vi "reward_behavior_michelle_visjitter_conswinAdapt_enticefx_TSLog_VF.vi"() -> ()   [LabVIEW 2019]
doc: "The myRIO Project template acquires acceleration data from the onboard accelerometer and displays the changes of acceleration values in a waveform chart."
uses:
  <vilib>/myRIO/Common/Instrument Driver Framework/Utilities/typedefs/Generic FPGA Reference.ctl
  <vilib>/myRIO/Common/Instrument Driver Framework/Utilities/typedefs/myRIO v1.0 Reference.ctl
  <vilib>/myRIO/Common/Instrument Driver Framework/Utilities/typedefs/Hardware Version Enum.ctl
  <vilib>/myRIO/Common/Instrument Driver Framework/Utilities/typedefs/myRIO Generic Hardware Reference.ctl
  <vilib>/userdefined/High Color/nirio_resource_hc.ctl
  <vilib>/myRIO/Common/Instrument Driver Framework/Utilities/vis/Is FPGA Ref Available.vi
  <vilib>/myRIO/Common/Instrument Driver Framework/myRIO v1.0/Encoder/typedefs/Encoder Signal Mode.ctl
  <vilib>/myRIO/Common/Instrument Driver Framework/myRIO v1.0/Encoder/typedefs/Encoder Channels Enum.ctl
  <vilib>/myRIO/Instrument Drivers/Onboard IO/Encoder/typedefs/Encoder Reference.ctl
  <vilib>/myRIO/Instrument Drivers/Onboard IO/Encoder/Encoder.lvlib
  <vilib>/myRIO/Instrument Drivers/Onboard IO/Encoder/vis/Read.vi
  <vilib>/myRIO/Common/Instrument Driver Framework/myRIO v1.0/Encoder/typedefs/Encoder Configuration v1.0.ctl
  <vilib>/myRIO/Common/Instrument Driver Framework/myRIO v1.0/Encoder/vis/myRIO v1.1 Open Encoder.vi
  <vilib>/myRIO/Common/Instrument Driver Framework/myRIO v1.0/Encoder/vis/myRIO v1.0 Configure Encoder.vi
  <vilib>/myRIO/Instrument Drivers/Onboard IO/Encoder/vis/myRIO Encoder Open.xnode
  <vilib>/myRIO/Express VI/Onboard IO/Encoder/Encoder Express VI.xnode
  <vilib>/myRIO/Express VI/Onboard IO/DI/DI Express VI.xnode
  <vilib>/myRIO/Instrument Drivers/Onboard IO/DIO/vis/Read.vi
  <vilib>/myRIO/Instrument Drivers/Onboard IO/DIO/DIO.lvlib
  <vilib>/myRIO/Common/Instrument Driver Framework/myRIO v1.0/DIO/typedefs/DIO Channels Enum.ctl
  <vilib>/myRIO/Common/Instrument Driver Framework/myRIO v1.0/DIO/typedefs/DIO Channels List.ctl
  <vilib>/myRIO/Instrument Drivers/Onboard IO/DIO/typedefs/DIO Reference.ctl
  <vilib>/myRIO/Instrument Drivers/Onboard IO/DIO/vis/myRIO DIO Open.xnode
  <vilib>/myRIO/Common/Instrument Driver Framework/myRIO v1.0/DIO/vis/myRIO v1.1 Open DIO.vi
  <vilib>/myRIO/Instrument Drivers/Onboard IO/DIO/vis/Write.vi
  <vilib>/myRIO/Express VI/Onboard IO/DO/DO Express VI.xnode
  <vilib>/myRIO/Common/Instrument Driver Framework/myRIO v1.0/Encoder/typedefs/Encoder Count Direction Enum.ctl
  <vilib>/Analysis/Matrix/Datatypes/RealMatrix.ctl
  <vilib>/Analysis/Matrix/NI_Matrix.lvlib
panel:
  out "GetVidFrame":i32
  out "VidTS":dbl[][](array[numeric])
  out "VidFrameClock":i32
  out "EntTS":dbl[][](array[numeric])
  out "TimeLag":dbl
  out "Lag2":dbl
  out "TestTime":dbl
  out "RewTS":dbl[][](array[numeric])
  out "ConsTS":dbl[][](array[numeric])
  out "LickTS":dbl[][](array[numeric])
  out "ContrastChoice":dbl
  out "Its":i32
  out "BurstCriteria":dbl
  out "LickBurst 2":bool
  out "LickBurst":bool
  out "Enticements":i32
  in  "Entice":bool
  out "Misses":i32
  out "GoAhead":bool
  out "TimeOutDuration":i32
  out "ActiveTime":dbl
  out "ConsumptionGo":bool=TRUE
  out "Consumption_Period":i32
  out "Watch_Display":bool=TRUE
  in  "Give reward":bool
  out "Timings":dbl[](array[numeric])
  out "ISI":dbl
  out "ISI start time":dbl
  out "Time_out":bool=TRUE
  out "Time since lick":dbl
  out "Time of last lick":dbl
  out "Rewarded trials":dbl[](array[numeric])
  out "Rewards":u16
  out "Active Trial":bool
  out "Array temp2":T1
  out "Stimuli Loaded":bool
  out "Stim_ID":dbl[](array[numeric])
  out "Reward_mat":dbl[](array[numeric])
  out "Reward":bool=TRUE
  out "Frame clock":i32
  out "Licks":u32
  out "Lick":bool
  out "Time":dbl
  out "Stop":bool
  in  "Frames to collect":u32
  out "Overflow?":bool
  out "Counter Value":i32
  out "Velocity":dbl
  out "Velocity Plot":dbl[](graph)
  out "Velocity array":dbl[](array[numeric])
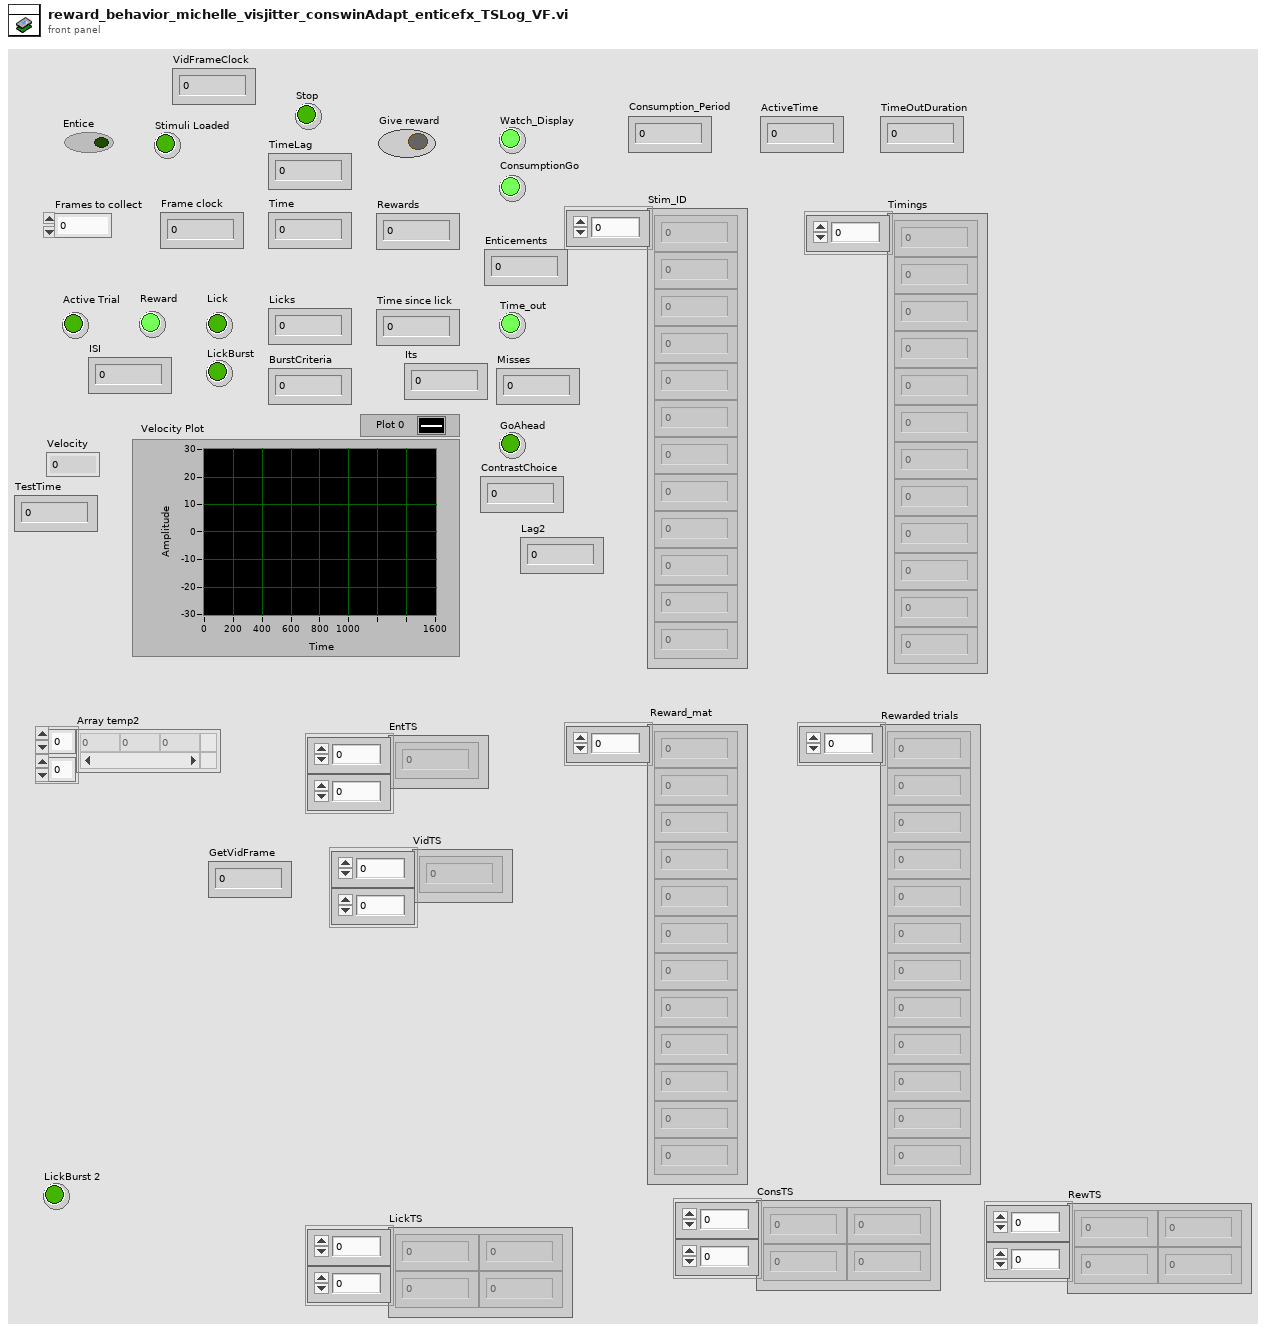
[diagram p1: front panel]
types:
  T1 = typedef "NI_Matrix.lvlib/RealMatrix.ctl" = dbl[][]
  T2 = typedef "Encoder.lvlib/Encoder Reference.ctl" = cluster{"myRIO Reference":T3, "Encoder Channels Enum":T7}
  T3 = typedef "myRIO Generic Hardware Reference.ctl" = cluster{"myRIO Model":T4, "myRIO Hardware Reference":T5}
  T4 = typedef "Hardware Version Enum.ctl" = enum16{"Unknown", "myRIO-1900", "myRIO-1950", "roboRIO", "NI ELVIS RIO CM", "ELVIS III"}
  T5 = typedef "myRIO v1.0 Reference.ctl" = cluster{"Generic FPGA Reference":T6, "Allow multiple opens":bool}
  T6 = typedef "Generic FPGA Reference.ctl" = refnum<k20>
  T7 = typedef "Encoder Channels Enum.ctl" = enum16{"Not Connected", "C/ENC0", "C/ENC1", "A/ENC", "A/ENC0", "A/ENC1", "A/ENC2", "A/ENC3", "A/ENC4", "A/ENC5", "A/ENC6", "A/ENC7", "A/ENC8", "A/ENC9", "B/ENC", "B/ENC0", "B/ENC1", "B/ENC2", "B/ENC3", "B/ENC4", "B/ENC5", "B/ENC6", "B/ENC7", "B/ENC8", "B/ENC9", "DIO/ENC0", "DIO/ENC1", "DIO/ENC2", "DIO/ENC3", "DIO/ENC4"}
  T8 = typedef "Encoder Signal Mode.ctl" = enum16{"Quadrature phase signal", "Step and direction signal"}
  T9 = typedef "nirio_resource_hc.ctl" = tag
  T10 = typedef "DIO.lvlib/DIO Reference.ctl" = cluster{"myRIO Reference":T3, "DIO Channels List":T11}
  T11 = typedef "DIO Channels List.ctl" = T12[]
  T12 = typedef "DIO Channels Enum.ctl" = enum16{"Not Connected", "C/DIO0", "C/DIO1", "C/DIO2", "C/DIO3", "C/DIO4", "C/DIO5", "C/DIO6", "C/DIO7", "A/DIO0", "A/DIO1", "A/DIO2", "A/DIO3", "A/DIO4", "A/DIO5", "A/DIO6", "A/DIO7", "A/DIO8", "A/DIO9", "A/DIO10", "A/DIO11", "A/DIO12", "A/DIO13", "A/DIO14", "A/DIO15", "A/DIO16", "A/DIO17", "A/DIO18", "A/DIO19", "B/DIO0", "B/DIO1", "B/DIO2", "B/DIO3", "B/DIO4", "B/DIO5", "B/DIO6", "B/DIO7", "B/DIO8", "B/DIO9", "B/DIO10", "B/DIO11", "B/DIO12", "B/DIO13", "B/DIO14", "B/DIO15", "B/DIO16", "B/DIO17", "B/DIO18", "B/DIO19", "LED0", "LED1", "LED2", "LED3", "Button0", "DIO/DIO0", "DIO/DIO1", "DIO/DIO2", "DIO/DIO3", "DIO/DIO4", "DIO/DIO5", "DIO/DIO6", "DIO/DIO7", "DIO/DIO8", "DIO/DIO9", "SPI/CS0", "SPI/CS1", "SPI/CS2", "SPI/CS3", "LED RADIO (Green)", "LED RADIO (Red)", "LED COMM (Green)", "LED COMM (Red)", "LED MODE (Green)", "LED MODE (Red)"}
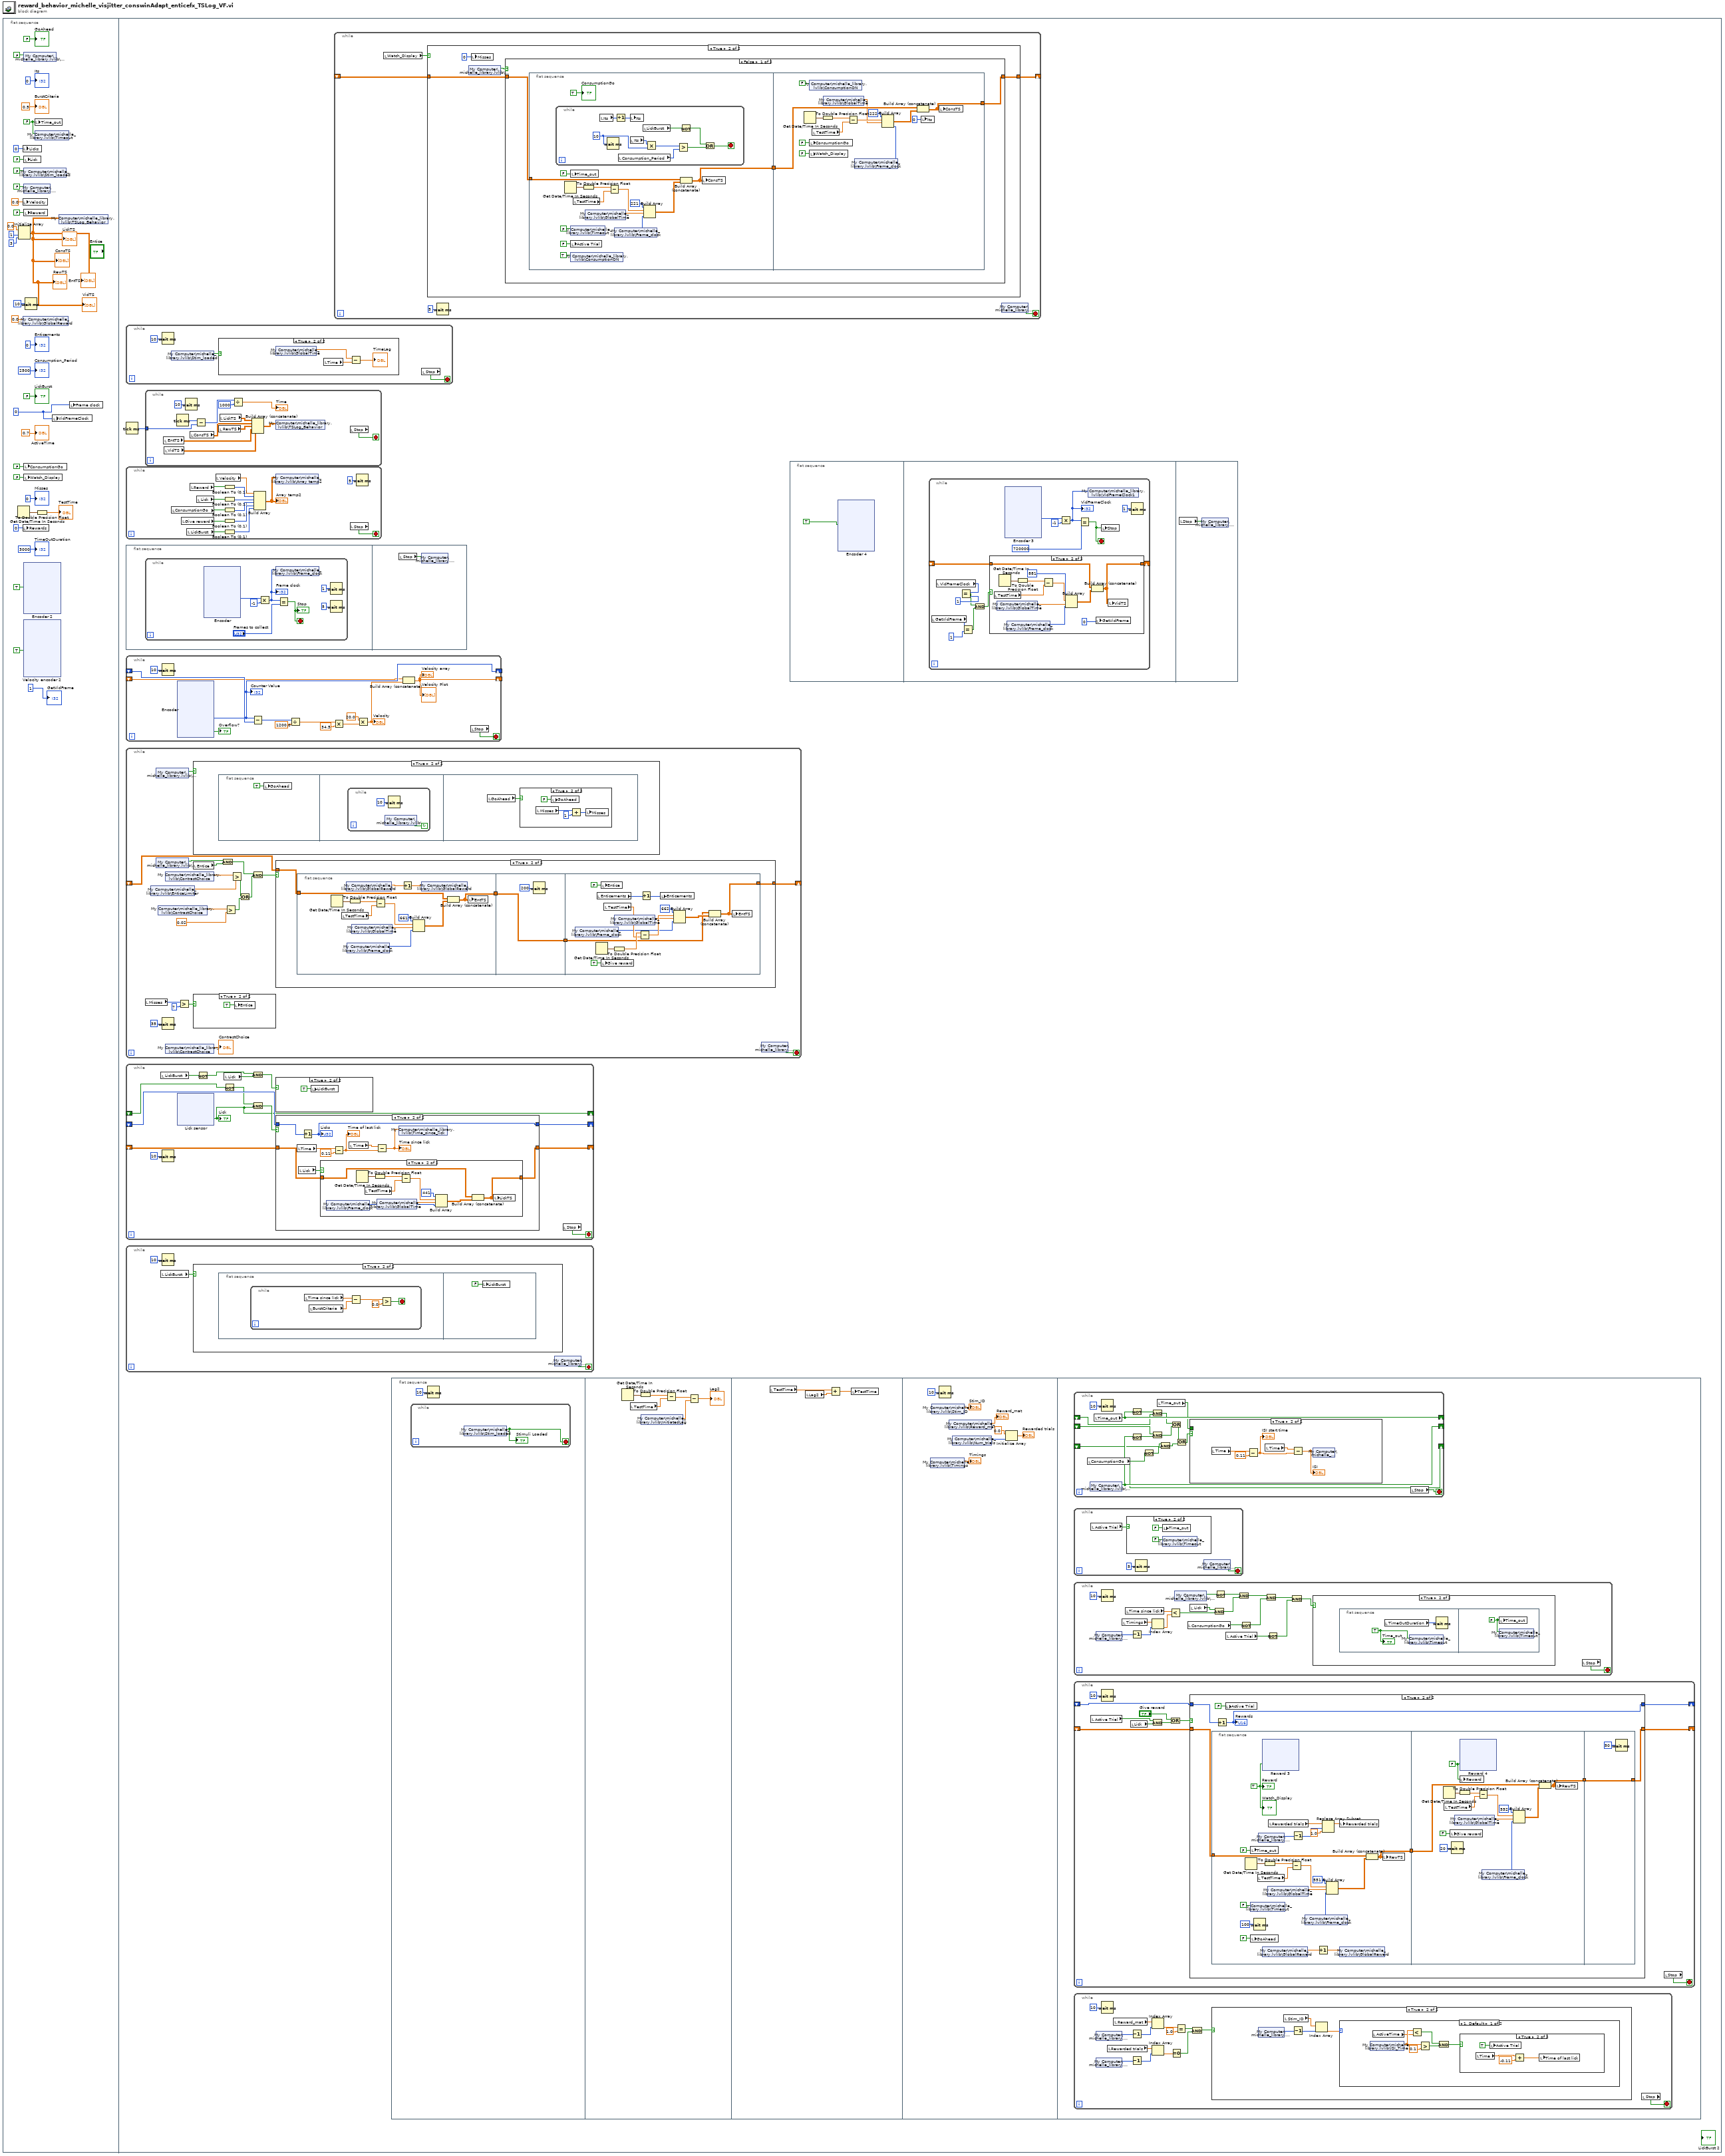
[diagram p0: block diagram]
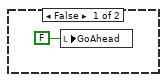
[diagram p7: hidden frame]
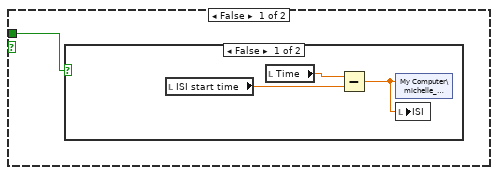
[diagram p13: hidden frame]
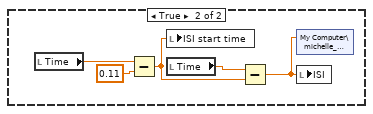
[diagram p14: hidden frame]
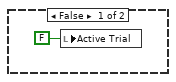
[diagram p15: hidden frame]
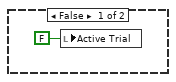
[diagram p16: hidden frame]
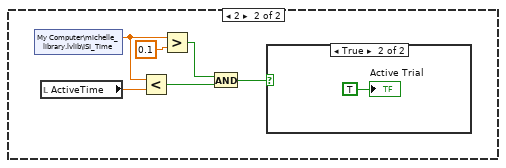
[diagram p17: hidden frame]
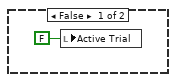
[diagram p18: hidden frame]
diagram:
  n1 = flat-sequence {
    frame #0 {
      w21 = FALSE ("Time_out")
      w3 = u32 0 ("Frames")
      n2 = Get Date/Time In Seconds() -> (seconds since 1Jan1904=w5:timestamp)
      n3 = Initialize Array(0.0, 1, 3) -> (w2:dbl[][])
      "LickTS" <- w2
      "ConsTS" <- w2
      "RewTS" <- w2
      "EntTS" <- w2
      "VidTS" <- w2
      n4 = local write "Licks"(u32 0 ("Licks")) -> ()
      n5 = local write "Velocity"(0.0 ("Velocity")) -> ()
      n6 = shared-variable "My Computer\\michelle_library.lvlib\\GlobalReward"(0.0) -> ()  [unwired: 1 in, 1 out]
      n7 = local write "Rewards"(u16 0 ("Rewards")) -> ()
      n8 = shared-variable "My Computer\\michelle_library.lvlib\\Display"(FALSE ("Display")) -> ()  [unwired: 1 in, 1 out]
      n9 = local write "Lick"(FALSE ("Lick")) -> ()
      n10 = shared-variable "My Computer\\michelle_library.lvlib\\Stim_loaded"(FALSE ("Stim_loaded")) -> ()  [unwired: 1 in, 1 out]
      n11 = shared-variable "My Computer\\michelle_library.lvlib\\Stop"(FALSE ("Stop")) -> ()  [unwired: 1 in, 1 out]
      n12 = local write "Reward"(FALSE ("Give reward")) -> ()
      n13 = local write "ConsumptionGo"(FALSE ("ConsumptionGo")) -> ()
      n14 = local write "Watch_Display"(FALSE ("Watch_Display")) -> ()
      n15 = xnode "Encoder 2"("Reset Counter"=TRUE) -> ()  [unwired: 1 in, 4 out]
      n16 = xnode "Velocity encoder 2"("Reset Counter"=TRUE) -> ()  [unwired: 1 in, 4 out]
      n17 = Wait (ms)(milliseconds to wait=u32 10) -> ()  [unwired: 1 out]
      n18 = local write "Time_out"(w21) -> ()
      n19 = shared-variable "My Computer\\michelle_library.lvlib\\Timeout"(w21) -> ()  [unwired: 1 in, 1 out]
      n20 = To Double Precision Float(number=w5) -> (double precision float=→"TestTime":dbl)
      n21 = local write "VidFrameClock"(w3) -> ()
      n22 = shared-variable "My Computer\\michelle_library.lvlib\\TSLog_Behavior"(w2) -> ()  [unwired: 1 in, 1 out]
      n23 = local write "Frame clock"(w3) -> ()
      "Consumption_Period" <- 2500
      "ActiveTime" <- 0.7
      "TimeOutDuration" <- 3000
      "GoAhead" <- FALSE
      "Misses" <- 0
      "Enticements" <- 0
      "LickBurst" <- FALSE
      "BurstCriteria" <- 0.5
      "Its" <- 0
      "GetVidFrame" <- 1
    }
    frame #1 {
      n24 = while {
        stop <- w248 stop-if-true
        n25 = Wait (ms)(milliseconds to wait=u32 10) -> ()  [unwired: 1 out]
        n26 = shared-variable "My Computer\\michelle_library.lvlib\\Stim_loaded"() -> (w249:bool)  [unwired: 1 in, 1 out]
        n27 = case shown="True" w249 {
          frame False {
          }
          frame True {
            n28 = shared-variable "My Computer\\michelle_library.lvlib\\GlobalTime"() -> (w250:dbl)  [unwired: 1 in, 1 out]
            n29 = local read "Time"() -> (w251:dbl)
            n30 = Subtract(x=w250, y=w251) -> (x-y=→"TimeLag":dbl)
          }
        }
        n31 = local read "Stop"() -> (w248:bool)
      }
      n32 = Tick Count (ms)() -> (millisecond timer value=w125:u32)
      n33 = while {
        stop <- w385 stop-if-true
        n34 = local read "ConsumptionGo"() -> (w383:bool)
        n35 = local read "Give reward"() -> (w382:bool)
        n36 = local read "LickBurst"() -> (w379:bool)
        n37 = local read "Reward"() -> (w390:bool)
        n38 = local read "Lick"() -> (w391:bool)
        n39 = local read "Velocity"() -> (w389:dbl)
        n40 = Boolean To (0,1)(Boolean=w390) -> (0, 1=w388:i16)
        n41 = Boolean To (0,1)(Boolean=w391) -> (0, 1=w387:i16)
        n42 = Boolean To (0,1)(Boolean=w383) -> (0, 1=w381:i16)
        n43 = Boolean To (0,1)(Boolean=w382) -> (0, 1=w380:i16)
        n44 = Boolean To (0,1)(Boolean=w379) -> (0, 1=w378:i16)
        n45 = Build Array(w389, w388, w387, w381, w380, w378) -> (w384:T1)
        "Array temp2" <- w384
        n46 = shared-variable "My Computer\\michelle_library.lvlib\\Array temp2"(w384) -> ()  [unwired: 1 in, 1 out]
        n47 = local read "Stop"() -> (w385:bool)
        n48 = Wait (ms)(milliseconds to wait=u32 5) -> ()  [unwired: 1 out]
      }
      n49 = flat-sequence {
        frame #0 {
          n50 = while {
            stop <- w634 stop-if-true
            n51 = xnode "Encoder"() -> ("Counter Value"=w638:i32)  [unwired: 2 in, 3 out]
            n52 = Multiply(x=w638, y=-1) -> (x*y=w633:i32)
            "Frame clock" <- w633
            n53 = shared-variable "My Computer\\michelle_library.lvlib\\Frame_clock"(w633) -> ()  [unwired: 1 in, 1 out]
            n54 = Equal?(x=w633, y="Frames to collect") -> (x = y?=w634:bool)
            "Stop" <- w634
            n55 = Wait (ms)(milliseconds to wait=u32 1) -> ()  [unwired: 1 out]
            n56 = Wait (ms)(milliseconds to wait=u32 5) -> ()  [unwired: 1 out]
          }
        }
        frame #1 {
          n57 = local read "Stop"() -> (w686:bool)
          n58 = shared-variable "My Computer\\michelle_library.lvlib\\Stop"(w686) -> ()  [unwired: 1 in, 1 out]
        }
      }
      n59 = while {
        shift-right: [w773] -> _
        shift-left: _ -> [w774]
        shift-right: [w765] -> _
        shift-left: _ -> [w764]
        stop <- w763 stop-if-true
        n60 = Wait (ms)(milliseconds to wait=u32 10) -> ()  [unwired: 1 out]
        n61 = xnode "Encoder"() -> ("Counter Value"=w773:i32, "Overflow?"=→"Overflow?":bool)  [unwired: 2 in, 2 out]
        "Counter Value" <- w773
        n62 = Subtract(x=w773, y=w774) -> (x-y=w766:i32)
        n63 = Divide(x=w766, y=1200.0 ("600")) -> (x/y=w771:dbl)
        n64 = Multiply(x=w771, y=34.5) -> (x*y=w769:dbl)
        n65 = Multiply(x=20.0, y=w769) -> (x*y=w767:dbl)
        "Velocity" <- w767
        n66 = Build Array (concatenate)(w764, w767) -> (w765:dbl[])
        "Velocity Plot" <- w765
        "Velocity array" <- w765
        n67 = local read "Stop"() -> (w763:bool)
      }
      n68 = while {
        shift-right: [w268] -> _
        shift-left: _ -> [w269]
        stop <- w281 stop-if-true
        n69 = local read "Misses"() -> (w279:i32)
        n70 = shared-variable "My Computer\\michelle_library.lvlib\\EnticeLimiter"() -> (w267:dbl)  [unwired: 1 in, 1 out]
        n71 = shared-variable "My Computer\\michelle_library.lvlib\\Display"() -> (w280:bool)  [unwired: 1 in, 1 out]
        n72 = shared-variable "My Computer\\michelle_library.lvlib\\Display"() -> (w276:bool)  [unwired: 1 in, 1 out]
        n73 = shared-variable "My Computer\\michelle_library.lvlib\\ContrastChoice"() -> (w263:dbl)  [unwired: 1 in, 1 out]
        n74 = Wait (ms)(milliseconds to wait=35) -> ()  [unwired: 1 out]
        n75 = shared-variable "My Computer\\michelle_library.lvlib\\ContrastChoice"() -> (w272:dbl)  [unwired: 1 in, 1 out]
        n76 = shared-variable "My Computer\\michelle_library.lvlib\\ContrastChoice"() -> (→"ContrastChoice":dbl)  [unwired: 1 in, 1 out]
        n77 = Greater?(x=w279, y=7) -> (0:w277:bool)
        n78 = case shown="True" w280 {
          frame False {
            n79 = local write "GoAhead"(FALSE) -> ()
          }
          frame True {
            n80 = flat-sequence {
              frame #0 {
                n81 = local write "GoAhead"(TRUE) -> ()
              }
              frame #1 {
                n82 = while {
                  stop <- w319 continue-if-true
                  n83 = shared-variable "My Computer\\michelle_library.lvlib\\Display"() -> (w319:bool)  [unwired: 1 in, 1 out]
                  n84 = Wait (ms)(milliseconds to wait=10) -> ()  [unwired: 1 out]
                }
              }
              frame #2 {
                n85 = local read "GoAhead"() -> (w320:bool)
                n86 = case shown="True" w320 {
                  frame False {
                  }
                  frame True {
                    n87 = local read "Misses"() -> (w324:i32)
                    n88 = local write "GoAhead"(FALSE) -> ()
                    n89 = Add(x=w324, y=1) -> (x+y=w322:i32)
                    n90 = local write "Misses"(w322) -> ()
                  }
                }
              }
            }
          }
        }
        n91 = local read "Entice"() -> (w275:bool)
        n92 = case shown="True" w277 {
          frame False {
          }
          frame True {
            n93 = local write "Entice"(TRUE) -> ()
          }
        }
        n94 = And(x=w276, y=w275) -> (x .and. y?=w273:bool)
        n95 = Greater?(x=w263, y=0.02) -> (0:w264:bool)
        n96 = Greater?(x=w272, y=w267) -> (0:w265:bool)
        n97 = Or(x=w265, y=w264) -> (x .or. y?=w266:bool)
        n98 = And(x=w273, y=w266) -> (x .and. y?=w271:bool)
        n99 = case shown="True" w271 {
          tunnel: w269 -> [w282 w286]
          tunnel: [w282 w283] -> w268
          frame False {
          }
          frame True {
            n100 = flat-sequence {
              tunnel: w286 -> [w289]
              tunnel: [w288] -> w285
              tunnel: w285 -> [w299]
              tunnel: [w299] -> w284
              tunnel: w284 -> [w303]
              tunnel: [w302] -> w283
              frame #0 {
                n101 = Get Date/Time In Seconds() -> (seconds since 1Jan1904=w296:timestamp)
                n102 = local read "TestTime"() -> (w291:dbl)
                n103 = shared-variable "My Computer\\michelle_library.lvlib\\GlobalReward"() -> (w298:dbl)  [unwired: 1 in, 1 out]
                n104 = shared-variable "My Computer\\michelle_library.lvlib\\Frame_clock"() -> (w287:u32)  [unwired: 1 in, 1 out]
                n105 = To Double Precision Float(number=w296) -> (double precision float=w295:dbl)
                n106 = shared-variable "My Computer\\michelle_library.lvlib\\GlobalTime"() -> (w290:dbl)  [unwired: 1 in, 1 out]
                n107 = Subtract(x=w295, y=w291) -> (x-y=w294:dbl)
                n108 = Increment(x=w298) -> (x+1=w297:dbl)
                n109 = Build Array(661, w294, w290, w287) -> (w293:T1)
                n110 = shared-variable "My Computer\\michelle_library.lvlib\\GlobalReward"(w297) -> ()  [unwired: 1 in, 1 out]
                n111 = Build Array (concatenate) ("Build Matrix")(w289, w293) -> (w288:T1)
                n112 = local write "EntTS"(w288) -> ()
              }
              frame #1 {
                n113 = Wait (ms)(milliseconds to wait=200) -> ()  [unwired: 1 out]
              }
              frame #2 {
                n114 = shared-variable "My Computer\\michelle_library.lvlib\\Frame_clock"() -> (w301:u32)  [unwired: 1 in, 1 out]
                n115 = Get Date/Time In Seconds() -> (seconds since 1Jan1904=w310:timestamp)
                n116 = local read "Enticements"() -> (w312:i32)
                n117 = local write "Entice"(FALSE) -> ()
                n118 = local write "Give reward"(TRUE) -> ()
                n119 = local read "TestTime"() -> (w304:dbl)
                n120 = To Double Precision Float(number=w310) -> (double precision float=w309:dbl)
                n121 = shared-variable "My Computer\\michelle_library.lvlib\\GlobalTime"() -> (w305:dbl)  [unwired: 1 in, 1 out]
                n122 = Subtract(x=w309, y=w304) -> (x-y=w308:dbl)
                n123 = Increment(x=w312) -> (x+1=w311:i32)
                n124 = local write "Enticements"(w311) -> ()
                n125 = Build Array(662, w308, w305, w301) -> (w307:T1)
                n126 = Build Array (concatenate) ("Build Matrix")(w303, w307) -> (w302:T1)
                n127 = local write "EntTS"(w302) -> ()
              }
            }
          }
        }
        n128 = shared-variable "My Computer\\michelle_library.lvlib\\Stop"() -> (w281:bool)  [unwired: 1 in, 1 out]
      }
      n129 = while {
        shift-right: [w699] -> _
        shift-left: _ -> [w698]
        shift-right: [w693] -> _
        shift-left: _ -> [w696]
        shift-right: [w687] -> _
        shift-left: _ -> [w688]
        stop <- w697 stop-if-true
        n130 = local read "LickBurst"() -> (w690:bool)
        n131 = Wait (ms)(milliseconds to wait=u32 10) -> ()  [unwired: 1 out]
        n132 = xnode "Lick sensor"() -> ("C/DIO1 (DIO1)"=w693:bool)  [unwired: 1 in, 1 out]
        "Lick" <- w693
        n133 = Not(x=w690) -> (.not. x?=w689:bool)
        n134 = Not(x=w696) -> (.not. x?=w695:bool)
        n135 = local read "Lick"() -> (w691:bool)
        n136 = And(x=w689, y=w691) -> (x .and. y?=w692:bool)
        n137 = And(x=w695, y=w693) -> (x .and. y?=w694:bool)
        n138 = case shown="True" w692 {
          frame False {
          }
          frame True {
            n139 = local write "LickBurst"(TRUE) -> ()
          }
        }
        n140 = case shown="True" w694 {
          tunnel: [w706 w716] -> w699
          tunnel: w698 -> [w706 w715]
          tunnel: w688 -> [w702 w707]
          tunnel: [w702 w709] -> w687
          frame False {
            n141 = local read "Time of last lick"() -> (w704:dbl)
            n142 = local read "Time"() -> (w705:dbl)
            n143 = Subtract(x=w705, y=w704) -> (x-y=w703:dbl)
            n144 = shared-variable "My Computer\\michelle_library.lvlib\\Time_since_lick"(w703) -> ()  [unwired: 1 in, 1 out]
            n145 = local write "Time since lick"(w703) -> ()
          }
          frame True {
            n146 = local read "Time"() -> (w712:dbl)
            n147 = local read "Lick"() -> (w708:bool)
            n148 = Increment(x=w715) -> (x+1=w716:u32)
            "Licks" <- w716
            n149 = case shown="True" w708 {
              tunnel: w707 -> [w717 w723]
              tunnel: [w717 w722] -> w709
              frame False {
              }
              frame True {
                n150 = shared-variable "My Computer\\michelle_library.lvlib\\Frame_clock"() -> (w718:u32)  [unwired: 1 in, 1 out]
                n151 = Get Date/Time In Seconds() -> (seconds since 1Jan1904=w725:timestamp)
                n152 = local read "TestTime"() -> (w720:dbl)
                n153 = To Double Precision Float(number=w725) -> (double precision float=w721:dbl)
                n154 = shared-variable "My Computer\\michelle_library.lvlib\\GlobalTime"() -> (w719:dbl)  [unwired: 1 in, 1 out]
                n155 = Subtract(x=w721, y=w720) -> (x-y=w726:dbl)
                n156 = Build Array(441, w726, w719, w718) -> (w727:T1)
                n157 = Build Array (concatenate) ("Build Matrix")(w723, w727) -> (w722:T1)
                n158 = local write "LickTS"(w722) -> ()
              }
            }
            n159 = Subtract(x=w712, y=0.11) -> (x-y=w710:dbl)
            "Time of last lick" <- w710
            n160 = local read "Time"() -> (w714:dbl)
            n161 = Subtract(x=w714, y=w710) -> (x-y=w713:dbl)
            "Time since lick" <- w713
            n162 = shared-variable "My Computer\\michelle_library.lvlib\\Time_since_lick"(w713) -> ()  [unwired: 1 in, 1 out]
          }
        }
        n163 = local read "Stop"() -> (w697:bool)
      }
      n164 = while {
        stop <- w255 stop-if-true
        n165 = local read "LickBurst"() -> (w253:bool)
        n166 = Wait (ms)(milliseconds to wait=u32 10) -> ()  [unwired: 1 out]
        n167 = case shown="True" w253 {
          frame False {
          }
          frame True {
            n168 = flat-sequence {
              frame #0 {
                n169 = while {
                  stop <- w258 stop-if-true
                  n170 = local read "Time since lick"() -> (w259:dbl)
                  n171 = local read "BurstCriteria"() -> (w260:dbl)
                  n172 = Subtract(x=w259, y=w260) -> (x-y=w256:dbl)
                  n173 = Greater?(x=w256, y=0.0) -> (0:w258:bool)
                }
              }
              frame #1 {
                n174 = local write "LickBurst"(FALSE) -> ()
              }
            }
          }
        }
        n175 = shared-variable "My Computer\\michelle_library.lvlib\\Stop"() -> (w255:bool)  [unwired: 1 in, 1 out]
      }
      n176 = while {
        tunnel: w125 -> [w834]
        stop <- w832 stop-if-true
        n177 = local read "EntTS"() -> (w824:dbl[][])
        n178 = local read "VidTS"() -> (w823:dbl[][])
        n179 = Tick Count (ms)() -> (millisecond timer value=w835:u32)
        n180 = Wait (ms)(milliseconds to wait=u32 10) -> ()  [unwired: 1 out]
        n181 = local read "ConsTS"() -> (w827:dbl[][])
        n182 = Subtract(x=w835, y=w834) -> (x-y=w831:u32)
        n183 = local read "RewTS"() -> (w826:dbl[][])
        n184 = local read "LickTS"() -> (w828:dbl[][])
        n185 = Divide(x=w831, y=u32 1000) -> (x/y=→"Time":dbl)
        n186 = Build Array (concatenate) ("Build Matrix")(w828, w827, w826, w824, w823) -> (w825:T1)
        n187 = shared-variable "My Computer\\michelle_library.lvlib\\TSLog_Behavior"(w825) -> ()  [unwired: 1 in, 1 out]
        n188 = local read "Stop"() -> (w832:bool)
      }
      n189 = while {
        shift-right: [w325] -> _
        shift-left: _ -> [w326]
        stop <- w329 stop-if-true
        n190 = local read "Watch_Display"() -> (w328:bool)
        n191 = case shown="True" w328 {
          tunnel: w326 -> [w330 w332]
          tunnel: [w330 w331] -> w325
          frame False {
          }
          frame True {
            n192 = shared-variable "My Computer\\michelle_library.lvlib\\Display"() -> (w334:bool)  [unwired: 1 in, 1 out]
            n193 = local write "Misses"(0) -> ()
            n194 = case shown="False" w334 {
              tunnel: w332 -> [w337 w377]
              tunnel: [w335 w377] -> w331
              frame False {
                n195 = flat-sequence {
                  tunnel: w337 -> [w341]
                  tunnel: [w340] -> w336
                  tunnel: w336 -> [w367]
                  tunnel: [w366] -> w335
                  frame #0 {
                    n196 = while {
                      stop <- w356 stop-if-true
                      w357 = 10
                      n197 = local read "Its"() -> (w361:i32)
                      n198 = Wait (ms)(milliseconds to wait=w357) -> ()  [unwired: 1 out]
                      n199 = Increment(x=w361) -> (x+1=w360:i32)
                      n200 = local read "Consumption_Period"() -> (w354:i32)
                      n201 = local write "Its"(w360) -> ()
                      n202 = local read "Its"() -> (w358:i32)
                      n203 = local read "LickBurst"() -> (w362:bool)
                      n204 = Multiply(x=w358, y=w357) -> (x*y=w355:i32)
                      n205 = Greater?(x=w355, y=w354) -> (0:w353:bool)
                      n206 = Not(x=w362) -> (.not. x?=w359:bool)
                      n207 = Or(x=w359, y=w353) -> (x .or. y?=w356:bool)
                    }
                    n208 = Get Date/Time In Seconds() -> (seconds since 1Jan1904=w346:timestamp)
                    n209 = local write "Time_out"(FALSE) -> ()
                    n210 = shared-variable "My Computer\\michelle_library.lvlib\\Timeout"(FALSE) -> ()  [unwired: 1 in, 1 out]
                    n211 = local write "Active Trial"(FALSE) -> ()
                    n212 = shared-variable "My Computer\\michelle_library.lvlib\\ConsumptionON"(TRUE) -> ()  [unwired: 1 in, 1 out]
                    n213 = local read "TestTime"() -> (w343:dbl)
                    n214 = To Double Precision Float(number=w346) -> (double precision float=w344:dbl)
                    n215 = shared-variable "My Computer\\michelle_library.lvlib\\GlobalTime"() -> (w339:dbl)  [unwired: 1 in, 1 out]
                    n216 = Subtract(x=w344, y=w343) -> (x-y=w347:dbl)
                    n217 = shared-variable "My Computer\\michelle_library.lvlib\\Frame_clock"() -> (w338:u32)  [unwired: 1 in, 1 out]
                    n218 = Build Array(221, w347, w339, w338) -> (w342:T1)
                    n219 = Build Array (concatenate) ("Build Matrix")(w341, w342) -> (w340:T1)
                    n220 = local write "ConsTS"(w340) -> ()
                    "ConsumptionGo" <- TRUE
                  }
                  frame #1 {
                    n221 = Get Date/Time In Seconds() -> (seconds since 1Jan1904=w371:timestamp)
                    n222 = shared-variable "My Computer\\michelle_library.lvlib\\ConsumptionON"(FALSE) -> ()  [unwired: 1 in, 1 out]
                    n223 = local write "ConsumptionGo"(FALSE ("ConsumptionGo")) -> ()
                    n224 = local write "Watch_Display"(FALSE ("Watch_Display")) -> ()
                    n225 = local read "TestTime"() -> (w368:dbl)
                    n226 = To Double Precision Float(number=w371) -> (double precision float=w369:dbl)
                    n227 = shared-variable "My Computer\\michelle_library.lvlib\\GlobalTime"() -> (w364:dbl)  [unwired: 1 in, 1 out]
                    n228 = Subtract(x=w369, y=w368) -> (x-y=w372:dbl)
                    n229 = shared-variable "My Computer\\michelle_library.lvlib\\Frame_clock"() -> (w363:u32)  [unwired: 1 in, 1 out]
                    n230 = Build Array(222, w372, w364, w363) -> (w365:T1)
                    n231 = Build Array (concatenate) ("Build Matrix")(w367, w365) -> (w366:T1)
                    n232 = local write "Its"(0) -> ()
                    n233 = local write "ConsTS"(w366) -> ()
                  }
                }
              }
              frame True {
              }
            }
          }
        }
        n234 = Wait (ms)(milliseconds to wait=u32 5) -> ()  [unwired: 1 out]
        n235 = shared-variable "My Computer\\michelle_library.lvlib\\Stop"() -> (w329:bool)  [unwired: 1 in, 1 out]
      }
      n236 = flat-sequence {
        frame #0 {
          n237 = while {
            stop <- w393 stop-if-true
            n238 = shared-variable "My Computer\\michelle_library.lvlib\\Stim_loaded"() -> (w393:bool)  [unwired: 1 in, 1 out]
            "Stimuli Loaded" <- w393
          }
          n239 = Wait (ms)(milliseconds to wait=u32 10) -> ()  [unwired: 1 out]
        }
        frame #1 {
          n240 = Get Date/Time In Seconds() -> (seconds since 1Jan1904=w399:timestamp)
          n241 = local read "TestTime"() -> (w398:dbl)
          n242 = To Double Precision Float(number=w399) -> (double precision float=w397:dbl)
          n243 = shared-variable "My Computer\\michelle_library.lvlib\\InitiatedLag"() -> (w396:dbl)  [unwired: 1 in, 1 out]
          n244 = Subtract(x=w397, y=w398) -> (x-y=w394:dbl)
          n245 = Subtract(x=w394, y=w396) -> (x-y=→"Lag2":dbl)
        }
        frame #2 {
          n246 = local read "TestTime"() -> (w400:dbl)
          n247 = local read "Lag2"() -> (w401:dbl)
          n248 = Add(x=w400, y=w401) -> (x+y=w402:dbl)
          n249 = local write "TestTime"(w402) -> ()
        }
        frame #3 {
          n250 = shared-variable "My Computer\\michelle_library.lvlib\\Timings"() -> (→"Timings":dbl[])  [unwired: 1 in, 1 out]
          n251 = shared-variable "My Computer\\michelle_library.lvlib\\Stim_ID"() -> (→"Stim_ID":dbl[])  [unwired: 1 in, 1 out]
          n252 = Wait (ms)(milliseconds to wait=u32 10) -> ()  [unwired: 1 out]
          n253 = shared-variable "My Computer\\michelle_library.lvlib\\Reward_mat"() -> (→"Reward_mat":dbl[])  [unwired: 1 in, 1 out]
          n254 = shared-variable "My Computer\\michelle_library.lvlib\\Num_trials"() -> (w406:u32)  [unwired: 1 in, 1 out]
          n255 = Initialize Array(0.0 ("element"), w406) -> (→"Rewarded trials":dbl[])
        }
        frame #4 {
          n256 = while {
            shift-right: [w452] -> _
            shift-left: _ -> [w450]
            shift-right: [w448] -> _
            shift-left: _ -> [w447]
            shift-right: [w442] -> _
            shift-left: _ -> [w440]
            stop <- w453 stop-if-true
            n257 = local read "ConsumptionGo"() -> (w442:bool)
            n258 = shared-variable "My Computer\\michelle_library.lvlib\\Display"() -> (w448:bool)  [unwired: 1 in, 1 out]
            n259 = local read "Time_out"() -> (w452:bool)
            n260 = Wait (ms)(milliseconds to wait=u32 10) -> ()  [unwired: 1 out]
            n261 = Not(x=w452) -> (.not. x?=w451:bool)
            n262 = Not(x=w448) -> (.not. x?=w446:bool)
            n263 = Not(x=w442) -> (.not. x?=w443:bool)
            n264 = And(x=w451, y=w450) -> (x .and. y?=w445:bool)
            n265 = And(x=w447, y=w446) -> (x .and. y?=w441:bool)
            n266 = local read "Time_out"() -> (w449:bool)
            n267 = And(x=w440, y=w443) -> (x .and. y?=w439:bool)
            n268 = Or(x=w445, y=w441) -> (x .or. y?=w438:bool)
            n269 = Or(x=w438, y=w439) -> (x .or. y?=w437:bool)
            n270 = case shown="True" w437 {
              tunnel: w449 -> [w454 _]
              frame False {
                n271 = case shown="False" w454 {
                  frame False {
                    n272 = local read "ISI start time"() -> (w457:dbl)
                    n273 = local read "Time"() -> (w456:dbl)
                    n274 = Subtract(x=w456, y=w457) -> (x-y=w455:dbl)
                    n275 = shared-variable "My Computer\\michelle_library.lvlib\\ISI"(w455) -> ()  [unwired: 1 in, 1 out]
                    n276 = local write "ISI"(w455) -> ()
                  }
                  frame True {
                    n277 = local read "Time"() -> (w462:dbl)
                    n278 = Subtract(x=w462, y=0.11) -> (x-y=w459:dbl)
                    n279 = local write "ISI start time"(w459) -> ()
                    n280 = local read "Time"() -> (w460:dbl)
                    n281 = Subtract(x=w460, y=w459) -> (x-y=w458:dbl)
                    n282 = shared-variable "My Computer\\michelle_library.lvlib\\ISI"(w458) -> ()  [unwired: 1 in, 1 out]
                    n283 = local write "ISI"(w458) -> ()
                  }
                }
              }
              frame True {
                n284 = local read "Time"() -> (w467:dbl)
                n285 = Subtract(x=w467, y=0.11) -> (x-y=w464:dbl)
                "ISI start time" <- w464
                n286 = local read "Time"() -> (w465:dbl)
                n287 = Subtract(x=w465, y=w464) -> (x-y=w463:dbl)
                "ISI" <- w463
                n288 = shared-variable "My Computer\\michelle_library.lvlib\\ISI"(w463) -> ()  [unwired: 1 in, 1 out]
              }
            }
            n289 = local read "Stop"() -> (w453:bool)
          }
          n290 = while {
            stop <- w412 stop-if-true
            n291 = local read "Active Trial"() -> (w411:bool)
            n292 = case shown="True" w411 {
              frame False {
              }
              frame True {
                n293 = local write "Time_out"(FALSE) -> ()
                n294 = shared-variable "My Computer\\michelle_library.lvlib\\Timeout"(FALSE) -> ()  [unwired: 1 in, 1 out]
              }
            }
            n295 = Wait (ms)(milliseconds to wait=5) -> ()  [unwired: 1 out]
            n296 = shared-variable "My Computer\\michelle_library.lvlib\\Stop"() -> (w412:bool)  [unwired: 1 in, 1 out]
          }
          n297 = while {
            stop <- w433 stop-if-true
            n298 = shared-variable "My Computer\\michelle_library.lvlib\\Trial"() -> (w423:u32)  [unwired: 1 in, 1 out]
            n299 = Wait (ms)(milliseconds to wait=u32 10) -> ()  [unwired: 1 out]
            n300 = local read "Timings"() -> (w425:dbl[])
            n301 = local read "Time since lick"() -> (w432:dbl)
            n302 = Decrement(x=w423) -> (x-1=w422:u32)
            n303 = Index Array(array=w425, index=w422) -> (element=w424:dbl)
            n304 = Less?(x=w432, y=w424) -> (x < y?=w431:bool)
            n305 = shared-variable "My Computer\\michelle_library.lvlib\\Display"() -> (w428:bool)  [unwired: 1 in, 1 out]
            n306 = local read "ConsumptionGo"() -> (w420:bool)
            n307 = local read "Lick"() -> (w430:bool)
            n308 = And(x=w430, y=w431) -> (x .and. y?=w426:bool)
            n309 = Not(x=w428) -> (.not. x?=w427:bool)
            n310 = local read "Active Trial"() -> (w415:bool)
            n311 = And(x=w427, y=w426) -> (x .and. y?=w419:bool)
            n312 = Not(x=w420) -> (.not. x?=w421:bool)
            n313 = And(x=w419, y=w421) -> (x .and. y?=w417:bool)
            n314 = Not(x=w415) -> (.not. x?=w418:bool)
            n315 = And(x=w417, y=w418) -> (x .and. y?=w416:bool)
            n316 = case shown="True" w416 {
              frame False {
              }
              frame True {
                n317 = flat-sequence {
                  frame #0 {
                    w435 = TRUE
                    n318 = local read "TimeOutDuration"() -> (w434:i32)
                    n319 = shared-variable "My Computer\\michelle_library.lvlib\\Timeout"(w435) -> ()  [unwired: 1 in, 1 out]
                    n320 = Wait (ms)(milliseconds to wait=w434) -> ()  [unwired: 1 out]
                    "Time_out" <- w435
                  }
                  frame #1 {
                    w436 = FALSE ("Timeout")
                    n321 = local write "Time_out"(w436) -> ()
                    n322 = shared-variable "My Computer\\michelle_library.lvlib\\Timeout"(w436) -> ()  [unwired: 1 in, 1 out]
                  }
                }
              }
            }
            n323 = local read "Stop"() -> (w433:bool)
          }
          n324 = while {
            shift-right: [w514] -> _
            shift-left: _ -> [w513]
            shift-right: [w506] -> _
            shift-left: _ -> [w507]
            stop <- w516 stop-if-true
            n325 = local read "Active Trial"() -> (w511:bool)
            n326 = Wait (ms)(milliseconds to wait=u32 10) -> ()  [unwired: 1 out]
            n327 = local read "Lick"() -> (w512:bool)
            n328 = And(x=w511, y=w512) -> (x .and. y?=w510:bool)
            n329 = Or(x="Give reward", y=w510) -> (x .or. y?=w509:bool)
            n330 = case shown="True" w509 {
              tunnel: [w518 w525] -> w514
              tunnel: w513 -> [w518 w524]
              tunnel: w507 -> [w517 w522]
              tunnel: [w517 w521] -> w506
              frame False {
              }
              frame True {
                n331 = flat-sequence {
                  tunnel: w522 -> [w531]
                  tunnel: [w528] -> w519
                  tunnel: [w587] -> w520
                  tunnel: w519 -> [w585]
                  tunnel: [w631] -> w521
                  tunnel: w520 -> [w631]
                  frame #0 {
                    w546 = TRUE ("C/DIO0 (DIO0)")
                    n332 = Get Date/Time In Seconds() -> (seconds since 1Jan1904=w535:timestamp)
                    n333 = local write "Time_out"(FALSE) -> ()
                    n334 = shared-variable "My Computer\\michelle_library.lvlib\\Timeout"(FALSE) -> ()  [unwired: 1 in, 1 out]
                    n335 = local write "GoAhead"(FALSE) -> ()
                    n336 = Wait (ms)(milliseconds to wait=u32 100) -> ()  [unwired: 1 out]
                    n337 = local read "TestTime"() -> (w529:dbl)
                    n338 = shared-variable "My Computer\\michelle_library.lvlib\\Trial"() -> (w545:u32)  [unwired: 1 in, 1 out]
                    n339 = xnode "Reward 3"("C/DIO0 (DIO0)"=w546) -> ()  [unwired: 1 in, 1 out]
                    n340 = shared-variable "My Computer\\michelle_library.lvlib\\GlobalReward"() -> (w537:dbl)  [unwired: 1 in, 1 out]
                    n341 = To Double Precision Float(number=w535) -> (double precision float=w534:dbl)
                    n342 = shared-variable "My Computer\\michelle_library.lvlib\\GlobalTime"() -> (w527:dbl)  [unwired: 1 in, 1 out]
                    n343 = local read "Rewarded trials"() -> (w543:dbl[])
                    n344 = Subtract(x=w534, y=w529) -> (x-y=w533:dbl)
                    n345 = Decrement(x=w545) -> (x-1=w544:u32)
                    n346 = shared-variable "My Computer\\michelle_library.lvlib\\Frame_clock"() -> (w526:u32)  [unwired: 1 in, 1 out]
                    n347 = Increment(x=w537) -> (x+1=w536:dbl)
                    n348 = Replace Array Subset(array=w543, new element=1.0 ("new element/subarray"), index=w544) -> (w541:dbl[])
                    n349 = Build Array(551, w533, w527, w526) -> (w532:T1)
                    n350 = local write "Rewarded trials"(w541) -> ()
                    n351 = shared-variable "My Computer\\michelle_library.lvlib\\GlobalReward"(w536) -> ()  [unwired: 1 in, 1 out]
                    n352 = Build Array (concatenate) ("Build Matrix")(w531, w532) -> (w528:T1)
                    n353 = local write "RewTS"(w528) -> ()
                    "Reward" <- w546
                    "Watch_Display" <- w546
                  }
                  frame #1 {
                    w595 = FALSE ("C/DIO0 (DIO0)")
                    n354 = Get Date/Time In Seconds() -> (seconds since 1Jan1904=w592:timestamp)
                    n355 = local read "TestTime"() -> (w586:dbl)
                    n356 = local write "Give reward"(FALSE ("Give reward")) -> ()
                    n357 = Wait (ms)(milliseconds to wait=u32 20) -> ()  [unwired: 1 out]
                    n358 = shared-variable "My Computer\\michelle_library.lvlib\\GlobalTime"() -> (w584:dbl)  [unwired: 1 in, 1 out]
                    n359 = To Double Precision Float(number=w592) -> (double precision float=w591:dbl)
                    n360 = xnode "Reward 4"("C/DIO0 (DIO0)"=w595) -> ()  [unwired: 1 in, 1 out]
                    n361 = local write "Reward"(w595) -> ()
                    n362 = Subtract(x=w591, y=w586) -> (x-y=w590:dbl)
                    n363 = shared-variable "My Computer\\michelle_library.lvlib\\Frame_clock"() -> (w583:u32)  [unwired: 1 in, 1 out]
                    n364 = Build Array(552, w590, w584, w583) -> (w588:T1)
                    n365 = Build Array (concatenate) ("Build Matrix")(w585, w588) -> (w587:T1)
                    n366 = local write "RewTS"(w587) -> ()
                  }
                  frame #2 {
                    n367 = Wait (ms)(milliseconds to wait=u32 50) -> ()  [unwired: 1 out]
                  }
                }
                n368 = Increment(x=w524) -> (x+1=w525:u16)
                "Rewards" <- w525
                n369 = local write "Active Trial"(FALSE ("Active Trial")) -> ()
              }
            }
            n370 = local read "Stop"() -> (w516:bool)
          }
          n371 = while {
            stop <- w481 stop-if-true
            n372 = shared-variable "My Computer\\michelle_library.lvlib\\Trial"() -> (w477:u32)  [unwired: 1 in, 1 out]
            n373 = shared-variable "My Computer\\michelle_library.lvlib\\Trial"() -> (w473:u32)  [unwired: 1 in, 1 out]
            n374 = Wait (ms)(milliseconds to wait=u32 10) -> ()  [unwired: 1 out]
            n375 = local read "Rewarded trials"() -> (w474:dbl[])
            n376 = local read "Reward_mat"() -> (w476:dbl[])
            n377 = Decrement(x=w477) -> (x-1=w478:u32)
            n378 = Decrement(x=w473) -> (x-1=w472:u32)
            n379 = Index Array(array=w476, index=w478) -> (element=w479:dbl)
            n380 = Index Array(array=w474, index=w472) -> (element=w471:dbl)
            n381 = Equal To 0?(x=w471) -> (x = 0?=w470:bool)
            n382 = Equal?(x=w479, y=1.0) -> (x = y?=w469:bool)
            n383 = And(x=w469, y=w470) -> (x .and. y?=w468:bool)
            n384 = case shown="True" w468 {
              frame False {
                n385 = local write "Active Trial"(FALSE ("Active_trial")) -> ()
              }
              frame True {
                n386 = shared-variable "My Computer\\michelle_library.lvlib\\Trial"() -> (w484:u32)  [unwired: 1 in, 1 out]
                n387 = local read "Stim_ID"() -> (w486:dbl[])
                n388 = Decrement(x=w484) -> (x-1=w485:u32)
                n389 = Index Array(array=w486, index=w485) -> (element=w483:dbl)
                n390 = case shown="1, Default" w483 {
                  frame 1, Default {
                    n391 = shared-variable "My Computer\\michelle_library.lvlib\\ISI_Time"() -> (w492:dbl)  [unwired: 1 in, 1 out]
                    n392 = local read "ActiveTime"() -> (w487:dbl)
                    n393 = Less?(x=w492, y=w487) -> (x < y?=w490:bool)
                    n394 = Greater?(x=w492, y=0.1) -> (0:w489:bool)
                    n395 = And(x=w490, y=w489) -> (x .and. y?=w488:bool)
                    n396 = case shown="True" w488 {
                      frame False {
                        n397 = local write "Active Trial"(FALSE ("Active Trial")) -> ()
                      }
                      frame True {
                        n398 = local read "Time"() -> (w496:dbl)
                        n399 = local write "Active Trial"(TRUE ("Active Trial")) -> ()
                        n400 = Add(x=w496, y=-0.11) -> (x+y=w494:dbl)
                        n401 = local write "Time of last lick"(w494) -> ()
                      }
                    }
                  }
                  frame 2 {
                    n402 = shared-variable "My Computer\\michelle_library.lvlib\\ISI_Time"() -> (w502:dbl)  [unwired: 1 in, 1 out]
                    n403 = local read "ActiveTime"() -> (w498:dbl)
                    n404 = Less?(x=w502, y=w498) -> (x < y?=w500:bool)
                    n405 = Greater?(x=w502, y=0.1) -> (0:w501:bool)
                    n406 = And(x=w501, y=w500) -> (x .and. y?=w499:bool)
                    n407 = case shown="True" w499 {
                      frame False {
                        n408 = local write "Active Trial"(FALSE ("Active Trial")) -> ()
                      }
                      frame True {
                        "Active Trial" <- TRUE ("Active Trial")
                      }
                    }
                  }
                }
              }
            }
            n409 = local read "Stop"() -> (w481:bool)
          }
        }
      }
      n410 = flat-sequence {
        frame #0 {
          n411 = xnode "Encoder 4"("Reset Counter"=TRUE) -> ()  [unwired: 1 in, 4 out]
        }
        frame #1 {
          n412 = while {
            shift-right: [w179] -> _
            shift-left: _ -> [w180]
            stop <- w184 stop-if-true
            n413 = local read "GetVidFrame"() -> (w174:i32)
            n414 = local read "VidFrameClock"() -> (w178:i32)
            n415 = Equal?(x=w178, y=1) -> (x = y?=w177:bool)
            n416 = Equal?(x=w174, y=1) -> (x = y?=w173:bool)
            n417 = And(x=w177, y=w173) -> (x .and. y?=w176:bool)
            n418 = case shown="True" w176 {
              tunnel: w180 -> [w188 w191]
              tunnel: [w188 w190] -> w179
              frame False {
              }
              frame True {
                n419 = local read "TestTime"() -> (w197:dbl)
                n420 = shared-variable "My Computer\\michelle_library.lvlib\\GlobalTime"() -> (w194:dbl)  [unwired: 1 in, 1 out]
                n421 = Get Date/Time In Seconds() -> (seconds since 1Jan1904=w199:timestamp)
                n422 = shared-variable "My Computer\\michelle_library.lvlib\\Frame_clock"() -> (w195:u32)  [unwired: 1 in, 1 out]
                n423 = To Double Precision Float(number=w199) -> (double precision float=w198:dbl)
                n424 = Subtract(x=w198, y=w197) -> (x-y=w196:dbl)
                n425 = Build Array(881, w196, w194, w195) -> (w193:T1)
                n426 = Build Array (concatenate) ("Build Matrix")(w191, w193) -> (w190:T1)
                n427 = local write "GetVidFrame"(0) -> ()
                n428 = local write "VidTS"(w190) -> ()
              }
            }
            n429 = xnode "Encoder 3"() -> ("Counter Value"=w186:i32)  [unwired: 2 in, 3 out]
            n430 = Multiply(x=w186, y=-1) -> (x*y=w183:i32)
            "VidFrameClock" <- w183
            n431 = Equal?(x=w183, y=720000) -> (x = y?=w184:bool)
            n432 = shared-variable "My Computer\\michelle_library.lvlib\\VidFrameClock1"(w183) -> ()  [unwired: 1 in, 1 out]
            n433 = local write "Stop"(w184) -> ()
            n434 = Wait (ms)(milliseconds to wait=u32 1) -> ()  [unwired: 1 out]
          }
        }
        frame #2 {
          n435 = local read "Stop"() -> (w246:bool)
          n436 = shared-variable "My Computer\\michelle_library.lvlib\\Stop"(w246) -> ()  [unwired: 1 in, 1 out]
        }
      }
    }
  }
